vi "U64-Array to U8.vi"(10 "U64 Array":u64[](array[numeric])) -> (2 "Byte Array":u8[](array[numeric]))   [LabVIEW 2014, in "hse-misc.lvlib"]
doc: "Convert an array of U64 to an array of Bytes (U8)."
uses:
  hse-misc.lvlib
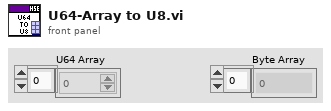
[diagram p1: front panel]
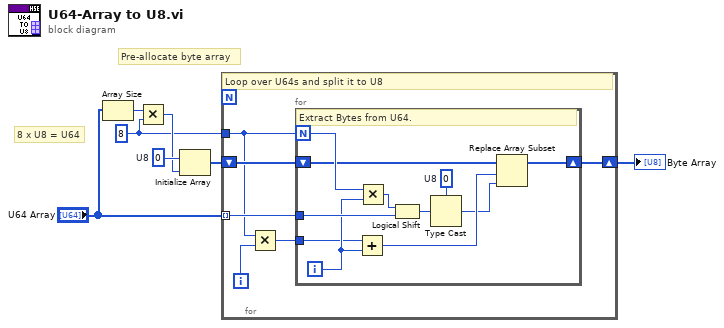
[diagram p0: block diagram]
diagram:
  w2 = 8 ("x")
  w7 = u8 0  # U8
  # "Pre-allocate byte array"
  # "8 x U8 = U64"
  n1 = Array Size(array="U64 Array") -> (size(s)=w4:i32)
  n2 = Multiply(x=w4, y=w2) -> (x*y=w3:i32)
  n3 = Initialize Array(w7, w3) -> (w6:u8[])
  n4 = for {
    tunnel: "U64 Array" -> [w13] mode=indexing
    tunnel: w2 -> [w11]
    shift-right: [w8] -> w1
    shift-left: w6 -> [w12]
    i -> [w10]
    # "Loop over U64s and split it to U8"
    n5 = Multiply(x=w11, y=w10) -> (x*y=w9:i32)
    n6 = for {
      N: w11 -> [w20]
      tunnel: w13 -> [w22]
      shift-right: [w18] -> w8
      shift-left: w12 -> [w19]
      tunnel: w9 -> [w16]
      i -> [w17]
      w24 = u8 0  # U8
      # "Extract Bytes from U64."
      n7 = Add(x=w16, y=w17) -> (x+y=w15:i32)
      n8 = Multiply(x=w20, y=w17) -> (x*y=w21:i32)
      n9 = Logical Shift(y=w21, x=w22) -> (x << y=w23:u64)
      n10 = Type Cast(type=w24, x=w23) -> (*(type *) &x=w14:u8)
      n11 = Replace Array Subset(array=w19, new element=w14, index=w15) -> (w18:u8[])
    }
  }
  "Byte Array" <- w1
